vi "Compute DistanceToBalls.vi"(6 "Target Width (in)":dbl=6.0 format="%#_13g", 8 "results":T1, 9 "Camera Type":T3, 11 "Image Src":T2) -> (0 "results out":T1, 3 "Image Dst Out":T2)   [LabVIEW 2019]
doc: "Using the camera lens information and the real world size of the target, use trig and ratios to determine the distance to the target. Also returns the location relative to the image center in a (-1 , 1) coordinate system that may be useful for steering the robot."
uses:
  Camera Types.ctl
  <vilib>/vision/Image Controls.llb/IMAQ Image.ctl
  Target Fields.ctl
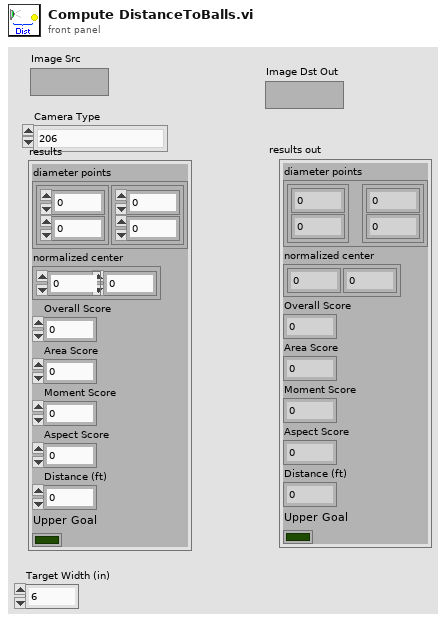
[diagram p1: front panel]
types:
  T1 = typedef "Target Fields.ctl" = cluster{"diameter points":cluster{"first point":cluster{"x":dbl, "y":dbl}, "projected point":cluster{"x":dbl, "y":dbl}}, "normalized center":cluster{"x":dbl, "y":dbl}, "Overall Score":dbl, "Area Score":dbl, "Moment Score":dbl, "Aspect Score":dbl, "Distance (ft)":dbl, "Upper Goal":bool}
  T2 = typedef "IMAQ Image.ctl" = refnum<image>
  T3 = typedef "Camera Types.ctl" = enum16{"206", "1011", "1013", "MS HD3000 square", "MS HD3000 640x480"}
  T4 = cluster{"first point":cluster{"x":dbl, "y":dbl}, "projected point":cluster{"x":dbl, "y":dbl}}
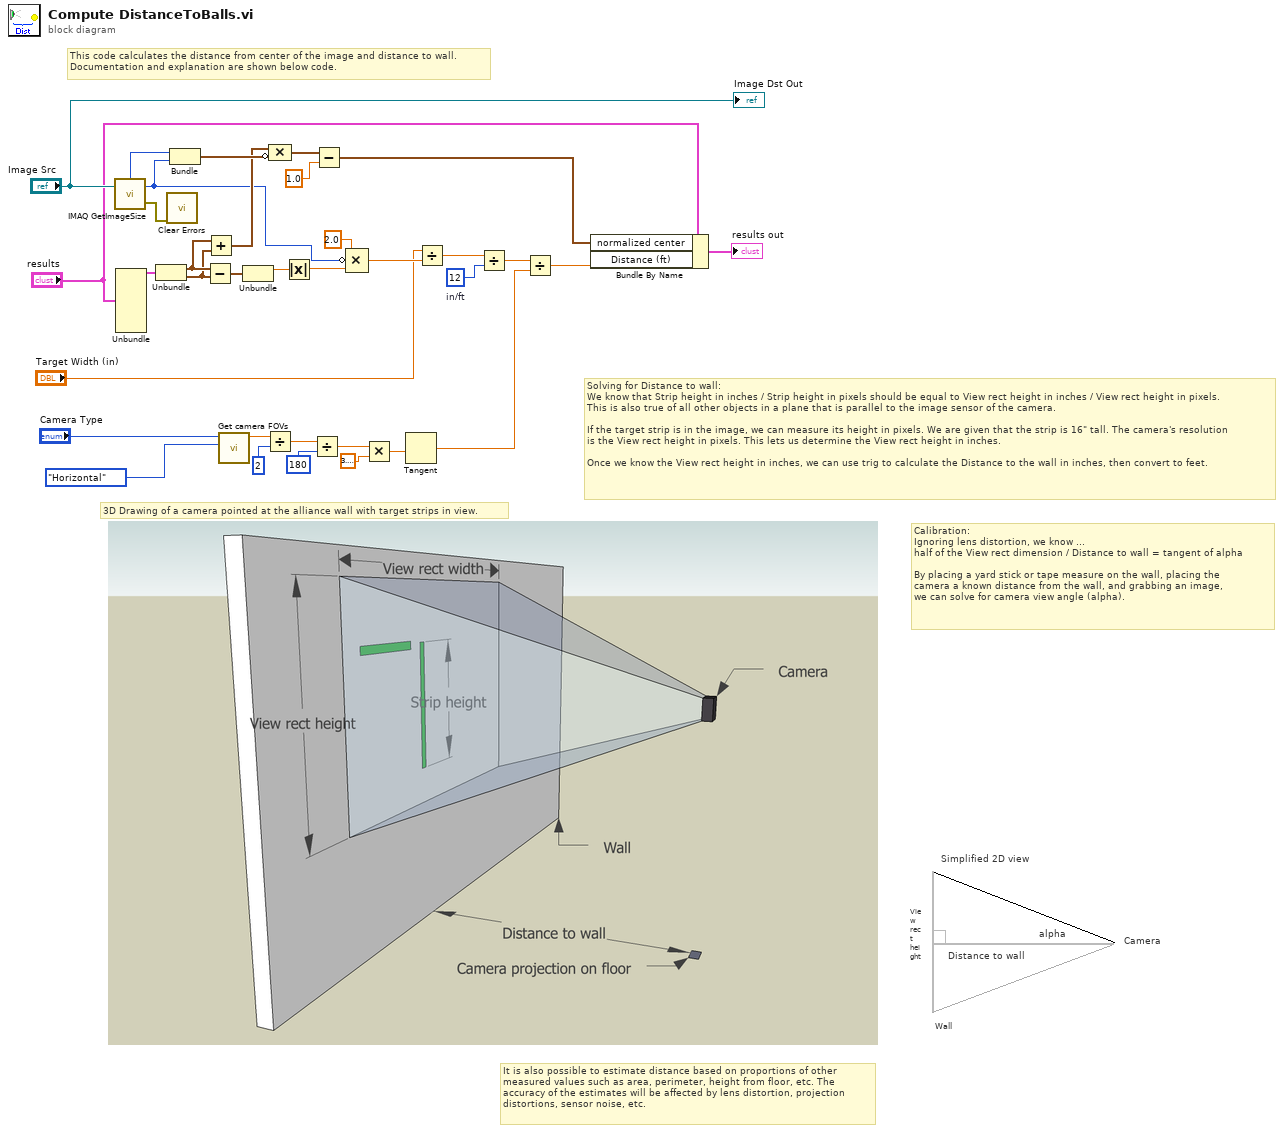
[diagram p0: block diagram]
diagram:
  w28 = 12  # in/ft
  # "It is also possible to estimate distance based on proportions of other\nmeasured values such as area, perimeter, height from floor, etc. The\naccuracy of the estimates will be affected by lens distortion, projection\ndistortions, sensor noise, etc."
  # "Wall"
  # "Camera"
  # "Simplified 2D view"
  # "Solving for Distance to wall:\nWe know that Strip height in inches / Strip height in pixels should be equal to View rect height in inches / View rect height in pixels.\nThis is also true of all other objects in a plane that is parallel to the image sensor of the camera.\n\nIf the target strip is in the image, we can measure its height in pixels. We are given that the strip is 16\" tall. The camera's resolution\nis the View rect height in pixels. This lets us determine the View rect height in inches.\n\nOnce we know the View rect height in inches, we can use trig to calculate the Distance to the wall in inches, then convert to feet."
  # "3D Drawing of a camera pointed at the alliance wall with target strips in view."
  # "Distance to wall"
  # "View rect height"
  # "alpha"
  # "Calibration:\nIgnoring lens distortion, we know ...\nhalf of the View rect dimension / Distance to wall = tangent of alpha\n\nBy placing a yard stick or tape measure on the wall, placing the\ncamera a known distance from the wall, and grabbing an image,\nwe can solve for camera view angle (alpha)."
  # "This code calculates the distance from center of the image and distance to wall.\nDocumentation and explanation are shown below code."
  n1 = call "IMAQ GetImageSize"("Image"="Image Src") -> ("Y Resolution"=w3:i32, "X Resolution"=w12:i32, "error out"=w21:errorcluster)  [unwired: 3 in]
  n2 = Unbundle("results") -> ("diameter points"=w11:T4)  [unwired: 7 out]
  n3 = Unbundle(w11) -> ("first point"=w7:cluster{"x":dbl, "y":dbl}, "projected point"=w6:cluster{"x":dbl, "y":dbl})
  n4 = call <vilib>:"Clear Errors.vi"("error in (no error)"=w21) -> ()  [unwired: 5 in, 2 out]
  n5 = Bundle("X Resolution"=w12, "Y Resolution"=w3) -> (w8:cluster{"X Resolution":i32, "Y Resolution":i32})  [unwired: 1 in]
  n6 = Subtract(x=w7, y=w6) -> (x-y=w17:cluster{"x":dbl, "y":dbl})
  n7 = Add(x=w7, y=w6) -> (x+y=w5:cluster{"x":dbl, "y":dbl})
  n8 = call "Get camera FOVs.vi"("Type"=enum16{"Horizontal", "Vertical", "Diagonal"}."Horizontal" ("Angle"), "Camera Type"="Camera Type") -> ("FOV"=w25:dbl)  [unwired: 8 in, 1 out]
  n9 = Unbundle(w17) -> ("x"=w16:dbl)  [unwired: 1 out]
  n10 = Divide(x=w25, y=2) -> (x/y=w31:dbl)
  n11 = Compound Arithmetic op=MULTIPLY(w5, invert w8) -> (w10:cluster{dbl, dbl})
  n12 = Absolute Value(x=w16) -> (abs(x)=w18:dbl)
  n13 = Divide(x=w31, y=180) -> (x/y=w30:dbl)
  n14 = Subtract(x=w10, y=1.0) -> (x-y=w9:cluster{dbl, dbl})
  n15 = Compound Arithmetic op=MULTIPLY(2.0, invert w3, w18) -> (w22:dbl)
  n16 = Multiply(x=w30, y=3.141592653589793) -> (x*y=w32:dbl)
  n17 = Tangent(1:w32) -> (0:w27:dbl)
  n18 = Divide(x="Target Width (in)", y=w22) -> (x/y=w19:dbl)
  n19 = Divide(x=w19, y=w28) -> (x/y=w26:dbl)
  n20 = Divide(x=w26, y=w27) -> (x/y=w13:dbl)
  n21 = Bundle By Name(cluster="results", "normalized center"=w9, "Distance (ft)"=w13) -> (→"results out":T1)
  "Image Dst Out" <- "Image Src"
